vi "Extract Time Stamp.vi"(8 "Error in":errorcluster, 11 "String":string) -> (0 "Error out":errorcluster, 2 "Time Stamp":timestamp, 3 "Error":bool)   [LabVIEW 2022 SP3]
uses:
  <vilib>/Utility/miscctls.llb/LVDateTimeRec.ctl
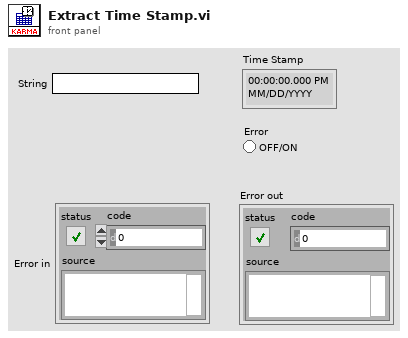
[diagram p1: front panel]
types:
  T1 = typedef "LVDateTimeRec.ctl" = cluster{"fractional second":dbl, "second":i32, "minute":i32, "hour":i32, "day of month":i32, "month":i32, "year":i32, "day of week":i32, "day of year":i32, "DST":i32}
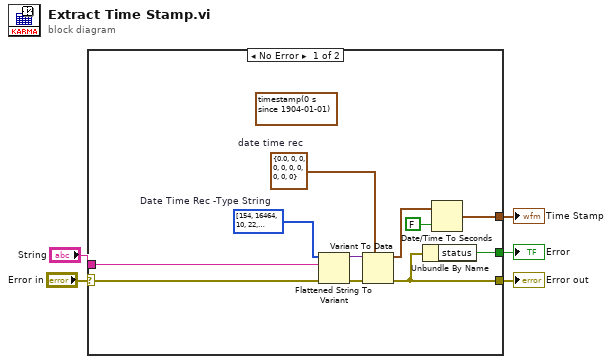
[diagram p0: block diagram]
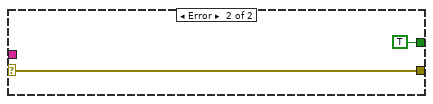
[diagram p2: hidden frame]
diagram:
  n1 = case shown="No Error" "Error in" {
    selector: "Error in" -> [w12 w18]
    tunnel: [w10 w18] -> w5
    tunnel: [w13 _] -> w4
    tunnel: "String" -> [w11 _]
    tunnel: [w9 TRUE ("status")] -> w1
    frame No Error {
      w6 = i16[] [154, 16464, 10, 22, 16394, 4454, 29281, 25460, 26991, 28257, 27680, 29541, 25455, 28260, 12, 16387, 1651, 25955, 28526, 25600, 12, 16387, 1645, 26990, 30068, 25856, 10, 16387, 1128, 28533, 29184, 18, 16387, 3172, 24953, 8303, 26144, 28015, 28276, 26624, 10, 16387, 1389, 28526, 29800, 10, 16387, 1145, 25953, 29184, 16, 16387, 2916, 24953, 8303, 26144, 30565, 25963, 16, 16387, 2916, 24953, 8303, 26144, 31077, 24946, 8, 16387, 836, 21332, 3428, 24948, 25888, 29801, 28005, 8306, 25955]  # Date Time Rec -Type String
      (unwired) timestamp(0 s since 1904-01-01) ("current time")
      w8 = T1 {"fractional second"=0.0, "second"=0, "minute"=0, "hour"=0, "day of month"=0, "month"=0, "year"=0, "day of week"=0, "day of year"=0, "DST"=0}  # date time rec
      n2 = Flattened String To Variant(4:w12, 6:w11, 7:w6) -> (0:w14:errorcluster, 3:w16:variant)
      n3 = Variant To Data(error in=w14, type=w8, Variant=w16) -> (data=w7:T1, error out=w10:errorcluster)
      n4 = Unbundle By Name(w10) -> ("status"=w9:bool)
      n5 = Date/Time To Seconds(1:FALSE ("is UTC (F)"), 2:w7) -> (0:w13:timestamp)
    }
    frame Error {
    }
  }
  "Error out" <- w5
  "Time Stamp" <- w4
  "Error" <- w1
